vi "Arc Turn.vi"(0 "Speed Setpoint (0-1)":dbl=0.3 format="%#_13g", 1 "Angle Radians (0 = Right)":dbl, 2 "Max Speed (TPS)":dbl=2500.0 format="%#_13g", 3 "Distance":dbl, 8 "Robot Width":dbl=24.0) -> (14 "Left Speed":dbl format="%#_13g", 16 "Right Speed":dbl format="%#_13g", 18 "Radius":dbl)   [LabVIEW 2015]
uses:
  Team900-VIs/Team900SwerveDrive/Team900SwerveDrive.lvlib
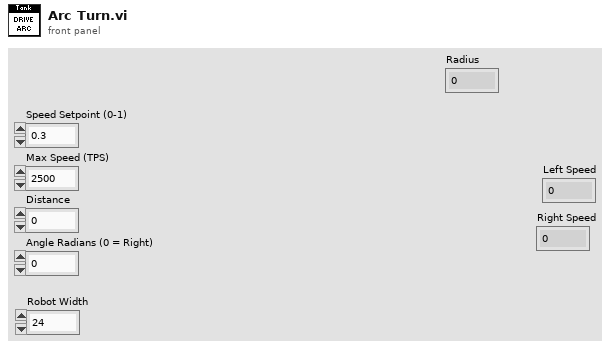
[diagram p1: front panel]
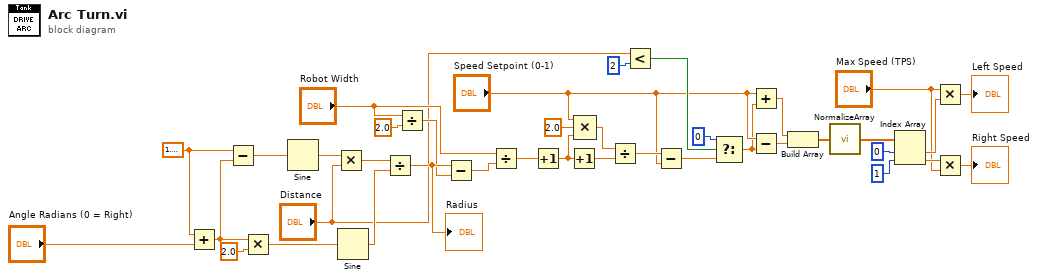
[diagram p0: block diagram]
diagram:
  w18 = 1.5707963267948966
  n1 = Add(x=w18, y="Angle Radians (0 = Right)") -> (x+y=w19:dbl)
  n2 = Subtract(x=w18, y=w19) -> (x-y=w38:dbl)
  n3 = Multiply(x=w19, y=2.0) -> (x*y=w34:dbl)
  n4 = Sine(x=w38) -> (sin(x)=w37:dbl)
  n5 = Multiply(x=w37, y="Distance") -> (x*y=w36:dbl)
  n6 = Sine(x=w34) -> (sin(x)=w33:dbl)
  n7 = Divide(x=w36, y=w33) -> (x/y=w32:dbl)
  "Radius" <- w32
  n8 = Divide(x="Robot Width", y=2.0) -> (x/y=w27:dbl)
  n9 = Subtract(x=w32, y=w27) -> (x-y=w31:dbl)
  n10 = Divide(x="Robot Width", y=w31) -> (x/y=w30:dbl)
  n11 = Increment(x=w30) -> (x+1=w8:dbl)
  n12 = Increment(x=w8) -> (x+1=w28:dbl)
  n13 = Compound Arithmetic op=MULTIPLY("Speed Setpoint (0-1)", 2.0 ("y"), w8) -> (w7:dbl)
  n14 = Divide(x=w7, y=w28) -> (x/y=w4:dbl)
  n15 = Less?(x="Distance", y=2) -> (x < y?=w6:bool)
  n16 = Subtract(x=w4, y="Speed Setpoint (0-1)") -> (x-y=w2:dbl)
  n17 = Select(t=0, s=w6, f=w2) -> (s? t:f=w1:dbl)
  n18 = Add(x="Speed Setpoint (0-1)", y=w1) -> (x+y=w10:dbl)
  n19 = Subtract(x="Speed Setpoint (0-1)", y=w1) -> (x-y=w11:dbl)
  n20 = Build Array(w10, w11) -> (w13:dbl[])
  n21 = call "NormalizeArray.vi"("array"=w13) -> ("normalized array"=w12:dbl[])
  n22 = Index Array(array=w12, index #1=0 ("index"), index #2=1 ("index")) -> (element #1=w16:dbl, element #2=w20:dbl)
  n23 = Multiply(x="Max Speed (TPS)", y=w16) -> (x*y=→"Left Speed":dbl)
  n24 = Multiply(x=w20, y="Max Speed (TPS)") -> (x*y=→"Right Speed":dbl)
